vi "Subvi Acquire Image.vi"(0 "ImgFile":string) -> (1 "ImgTaken":bool, 2 "ImgAbort":bool)   [LabVIEW 2012]
uses:
  ProSCI Global.vi
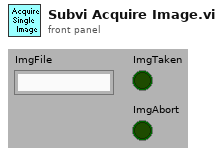
[diagram p1: front panel]
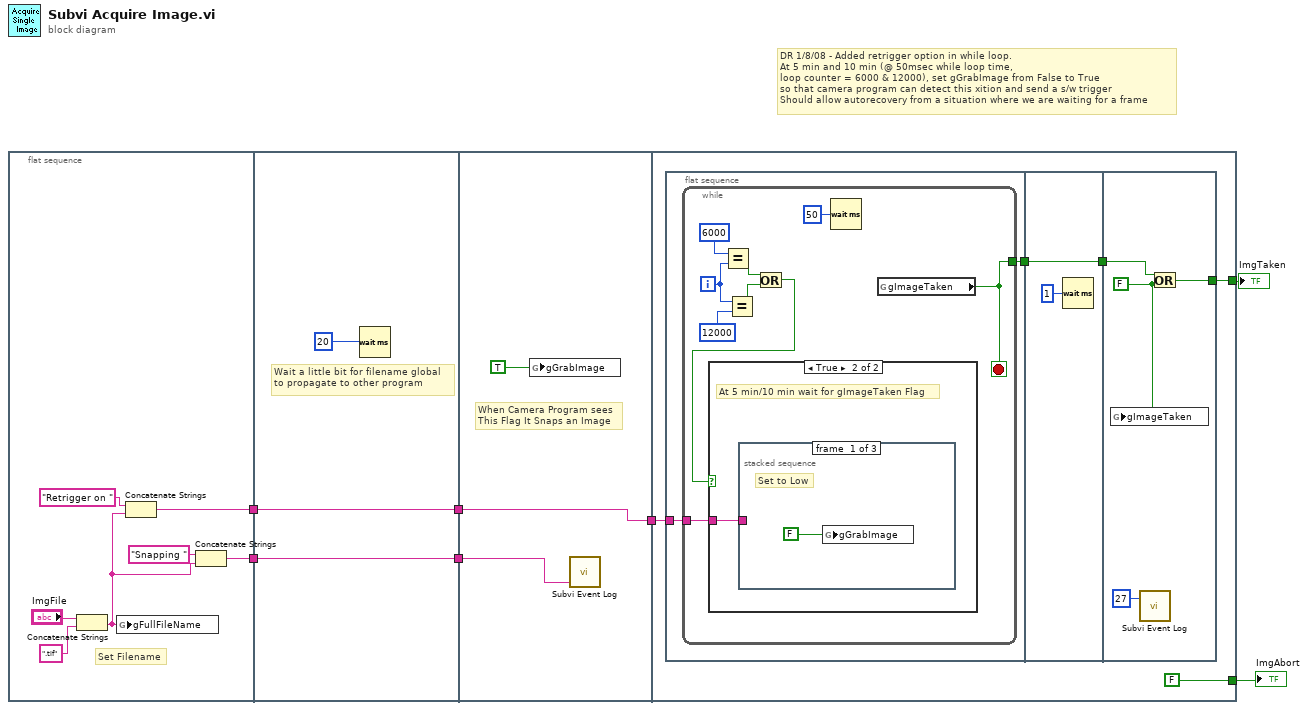
[diagram p0: block diagram]
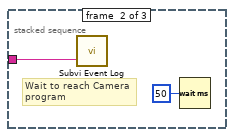
[diagram p3: hidden frame]
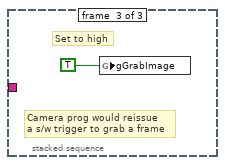
[diagram p4: hidden frame]
diagram:
  # "DR 1/8/08 - Added retrigger option in while loop.\nAt 5 min and 10 min (@ 50msec while loop time,\nloop counter = 6000 & 12000), set gGrabImage from False to True\nso that camera program can detect this xition and send a s/w trigger\nShould allow autorecovery from a situation where we are waiting for a frame"
  n1 = flat-sequence {
    tunnel: [w11] -> w3
    tunnel: [w8] -> w1
    tunnel: [w16] -> w4
    tunnel: w3 -> [w16]
    tunnel: [w15] -> w2
    tunnel: w1 -> [w15]
    tunnel: [w19] -> w5
    tunnel: w4 -> [w19]
    tunnel: w2 -> [w18]
    tunnel: [w23] -> w7
    tunnel: [FALSE] -> w6
    tunnel: w5 -> [w21]
    frame #0 {
      # "Set Filename"
      n2 = Concatenate Strings("ImgFile", ".tif" ("string")) -> (w9:string)
      n3 = global write "ProSCI Global.vi" "gFullFileName"(w9) -> ()
      n4 = Concatenate Strings("Retrigger on ", w9) -> (w11:string)
      n5 = Concatenate Strings("Snapping " ("string"), w9) -> (w8:string)
    }
    frame #1 {
      # "Wait a little bit for filename global\nto propagate to other program"
      n6 = Wait (ms)(milliseconds to wait=u32 20) -> ()  [unwired: 1 out]
    }
    frame #2 {
      # "When Camera Program sees\nThis Flag It Snaps an Image"
      n7 = global write "ProSCI Global.vi" "gGrabImage"(TRUE ("gGrabImage")) -> ()
      n8 = call "Subvi Event Log.vi"("CustomMessage"=w18) -> ()  [unwired: 1 in]
    }
    frame #3 {
      n9 = flat-sequence {
        tunnel: [w27] -> w24
        tunnel: w21 -> [w26]
        tunnel: [w42] -> w25
        tunnel: w24 -> [w42]
        tunnel: [w47] -> w23
        tunnel: w25 -> [w46]
        frame #0 {
          n10 = while {
            tunnel: [w35] -> w27
            tunnel: w26 -> [w28]
            i -> [w33]
            stop <- w35 stop-if-true
            n11 = Equal?(x=u32 6000 ("milliseconds to wait"), y=w33) -> (x = y?=w30:bool)
            n12 = Equal?(x=w33, y=u32 12000 ("milliseconds to wait")) -> (x = y?=w31:bool)
            n13 = Or(x=w30, y=w31) -> (x .or. y?=w29:bool)
            n14 = case shown="True" w29 {
              tunnel: w28 -> [_ w37]
              frame False {
              }
              frame True {
                # "At 5 min/10 min wait for gImageTaken Flag"
                n15 = stacked-sequence {
                  tunnel: w37 -> [_ w39 _]
                  frame #0 {
                    # "Set to Low"
                    n16 = global write "ProSCI Global.vi" "gGrabImage"(FALSE ("gGrabImage")) -> ()
                  }
                  frame #1 {
                    # "Wait to reach Camera\nprogram"
                    n17 = call "Subvi Event Log.vi"("CustomMessage"=w39) -> ()  [unwired: 1 in]
                    n18 = Wait (ms)(milliseconds to wait=u32 50) -> ()  [unwired: 1 out]
                  }
                  frame #2 {
                    # "Camera prog would reissue\na s/w trigger to grab a frame"
                    # "Set to high"
                    n19 = global write "ProSCI Global.vi" "gGrabImage"(TRUE ("gGrabImage")) -> ()
                  }
                }
              }
            }
            n20 = Wait (ms)(milliseconds to wait=u32 50) -> ()  [unwired: 1 out]
            n21 = global read "ProSCI Global.vi" "gImageTaken"() -> (w35:bool)
          }
        }
        frame #1 {
          n22 = Wait (ms)(milliseconds to wait=u32 1) -> ()  [unwired: 1 out]
        }
        frame #2 {
          w44 = FALSE ("y")
          n23 = global write "ProSCI Global.vi" "gImageTaken"(w44) -> ()
          n24 = call "Subvi Event Log.vi"("EventNum"=u32 27) -> ()  [unwired: 1 in]
          n25 = Or(x=w46, y=w44) -> (x .or. y?=w47:bool)
        }
      }
    }
  }
  "ImgAbort" <- w6
  "ImgTaken" <- w7
